vi "SRX_Config Voltage Output.vi"(8 "Error":errorcluster, 9 "Output Config":T1={"Invert?"=FALSE, "Neutral Mode"=enum."Override to Coast", "Deadband (-1to1)"=0.0, "Ramp Time Off to Full (S)"=0.0, "Peak  (-1to1)"={"Forward"=1.0, "Reverse"=-1.0}, "Nominal  (-1to1)"={"Forward"=0.0, "Reverse"=0.0}}, 11 "PhoenixMotorControlDevRef":T4={"DeviceStatus"={"status"=FALSE, "code"=0, "source"=""}, "Type"=enum."PWM", "PWM"={"PWM Channel"=enum."PWM 1", "DeadBand"={"Name"="", "maxPositivePwm"=0, "minPositivePwm"=0, "centerPwm"=0, "maxNegativePwm"=0, "minNegativePwm"=0, "angularRange"=0}}, "CAN"={"Device Number"=0, "SetOutput VI Ref"=variant(enum8{"Percent VBus", "Current", "Speed", "Position", "Voltage"} enum."Percent VBus"), "GetOutput VI Ref"=variant(refnum<k1> refnum), "Enable VI Ref"=variant(dbl 12.0), "Disable VI Ref"=variant(enum8{"Percent VBus", "Speed", "Position", "Slave", "Unchanged / Invalid", "Voltage Compensation", "Current", "Motion Profile"} enum."Percent VBus"), "Data"=variant}, "Invert"=FALSE, "DIO PWM"={"PWM \"Enable\" Channel"=enum."Invalid", "DIOChannel"=enum."Invalid", "PWM Rate"=0.0}}) -> (0 "Error Out":errorcluster, 3 "PhoenixMotorControlDevRef Out":T4={"DeviceStatus"={"status"=FALSE, "code"=0, "source"=""}, "Type"=enum."PWM", "PWM"={"PWM Channel"=enum."PWM 1", "DeadBand"={"Name"="", "maxPositivePwm"=0, "minPositivePwm"=0, "centerPwm"=0, "maxNegativePwm"=0, "minNegativePwm"=0, "angularRange"=0}}, "CAN"={"Device Number"=0, "SetOutput VI Ref"=variant(enum8{"Percent VBus", "Current", "Speed", "Position", "Voltage"} enum."Percent VBus"), "GetOutput VI Ref"=variant(refnum<k1> refnum), "Enable VI Ref"=variant(dbl 12.0), "Disable VI Ref"=variant(enum8{"Percent VBus", "Speed", "Position", "Slave", "Unchanged / Invalid", "Voltage Compensation", "Current", "Motion Profile"} enum."Percent VBus"), "Data"=variant}, "Invert"=FALSE, "DIO PWM"={"PWM \"Enable\" Channel"=enum."Invalid", "DIOChannel"=enum."Invalid", "PWM Rate"=0.0}})   [LabVIEW 2017]
uses:
  <vilib>/Rock Robotics/WPI/MotorControl/WPI_MotorControlDeviceRef.ctl
  <vilib>/Rock Robotics/WPI/MotorControl/WPI_MotorControlType.ctl
  <vilib>/Rock Robotics/SystemInterfaces/DIO/FPGA_DIOPWMChannel.ctl
  <vilib>/Rock Robotics/WPI/PWM/WPI_PWMDeadband.ctl
  <vilib>/Rock Robotics/SystemInterfaces/DIO/FPGA_DIOChannel.ctl
  TypeDefs SRX/Cluster_SRX_Config Voltage Output.ctl
  System Drivers/Phoenix-LabVIEW/Motor Controller/Controls/CTRE_Phoenix_MotorControl_NeutralMode.ctl
  TypeDefs SRX/Cluster_SRX_Forward and Reverse.ctl
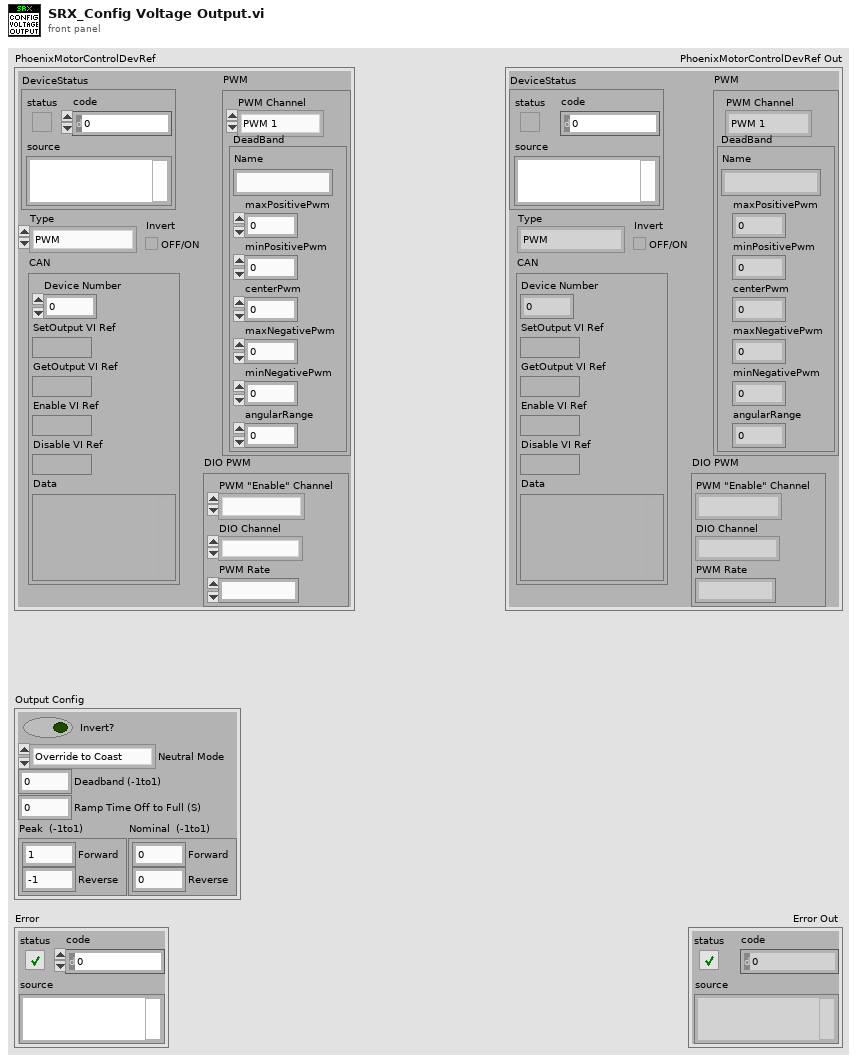
[diagram p1: front panel]
types:
  T1 = typedef "Cluster_SRX_Config Voltage Output.ctl" = cluster{"Invert?":bool, "Neutral Mode":T2, "Deadband (-1to1)":dbl, "Ramp Time Off to Full (S)":dbl, "Peak  (-1to1)":T3, "Nominal  (-1to1)":T3}
  T2 = typedef "CTRE_Phoenix_MotorControl_NeutralMode.ctl" = enum8{"EEPROMSetting", "Override to Coast", "Override to Brake"}
  T3 = typedef "Cluster_SRX_Forward and Reverse.ctl" = cluster{"Forward":dbl, "Reverse":dbl}
  T4 = typedef "WPI_MotorControlDeviceRef.ctl" = cluster{"DeviceStatus":errorcluster, "Type":T5, "PWM":cluster{"PWM Channel":T6, "DeadBand":T7}, "CAN":cluster{"Device Number":u8, "SetOutput VI Ref":variant, "GetOutput VI Ref":variant, "Enable VI Ref":variant, "Disable VI Ref":variant, "Data":variant}, "Invert":bool, "DIO PWM":cluster{"PWM \"Enable\" Channel":T6, "DIOChannel":T8, "PWM Rate":dbl}}
  T5 = typedef "WPI_MotorControlType.ctl" = enum16{"PWM", "CAN", "DIO PWM"}
  T6 = typedef "FPGA_DIOPWMChannel.ctl" = enum8{"PWM 0", "PWM 1", "PWM 2", "PWM 3", "PWM 4", "PWM 5", "PWM 6", "PWM 7", "PWM 8", "PWM 9", "PWM MXP 0", "PWM MXP 1", "PWM MXP 2", "PWM MXP 3", "PWM MXP 4", "PWM MXP 5", "PWM MXP 6", "PWM MXP 7", "PWM MXP 8", "PWM MXP 9", "Invalid"}
  T7 = typedef "WPI_PWMDeadband.ctl" = cluster{"Name":string, "maxPositivePwm":i32, "minPositivePwm":i32, "centerPwm":i32, "maxNegativePwm":i32, "minNegativePwm":i32, "angularRange":u16}
  T8 = typedef "FPGA_DIOChannel.ctl" = enum8{"DIO 0", "DIO 1", "DIO 2", "DIO 3", "DIO 4", "DIO 5", "DIO 6", "DIO 7", "DIO 8", "DIO 9", "DIO MXP 0", "DIO MXP 1", "DIO MXP 2", "DIO MXP 3", "DIO MXP 4", "DIO MXP 5", "DIO MXP 6", "DIO MXP 7", "DIO MXP 8", "DIO MXP 9", "DIO MXP 10", "DIO MXP 11", "DIO MXP 12", "DIO MXP 13", "DIO MXP 14", "DIO MXP 15", "SPI Port CS1", "SPI Port CS2", "SPI Port CS3", "SPI Port MISO", "SPI Port MOSI", "Invalid"}
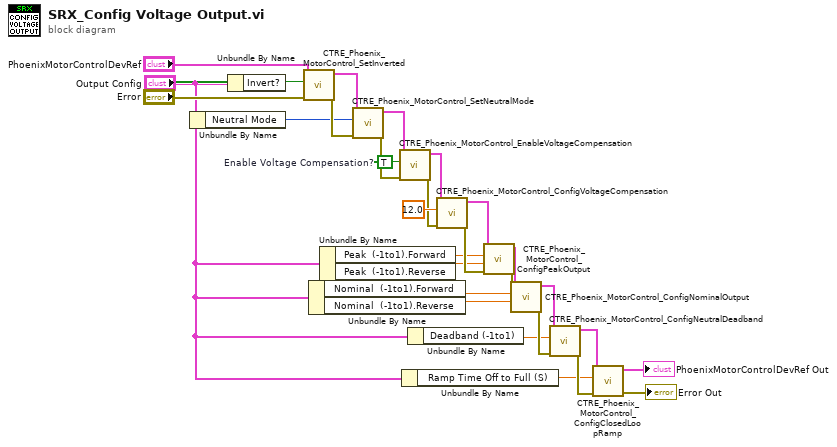
[diagram p0: block diagram]
diagram:
  w20 = TRUE  # Enable Voltage Compensation?
  n1 = Unbundle By Name("Output Config") -> ("Neutral Mode"=w8:T2)
  n2 = Unbundle By Name("Output Config") -> ("Invert?"=w9:bool)
  n3 = call "CTRE_Phoenix_MotorControl_SetInverted.vi"("error in (no error)"="Error", "Invert?"=w9, "PhoenixMotorControlDevRef"="PhoenixMotorControlDevRef") -> ("error out"=w11:errorcluster, "PhoenixMotorControlDevRef"=w27:T4)  [unwired: 7 in]
  n4 = Unbundle By Name("Output Config") -> ("Nominal  (-1to1).Forward"=w5:dbl, "Nominal  (-1to1).Reverse"=w4:dbl)
  n5 = Unbundle By Name("Output Config") -> ("Peak  (-1to1).Forward"=w6:dbl, "Peak  (-1to1).Reverse"=w7:dbl)
  n6 = call "CTRE_Phoenix_MotorControl_SetNeutralMode.vi"("error in (no error)"=w11, "Motor Control Neutral Mode"=w8, "PhoenixMotorControlDevRef"=w27) -> ("error out"=w12:errorcluster, "PhoenixMotorControlDevRef"=w26:T4)  [unwired: 7 in]
  n7 = call "CTRE_Phoenix_MotorControl_EnableVoltageCompensation.vi"("error in (no error)"=w12, "Enable Voltage Compensation?"=w20, "PhoenixMotorControlDevRef"=w26) -> ("error out"=w13:errorcluster, "PhoenixMotorControlDevRef"=w25:T4)  [unwired: 7 in]
  n8 = Unbundle By Name("Output Config") -> ("Ramp Time Off to Full (S)"=w1:dbl)
  n9 = Unbundle By Name("Output Config") -> ("Deadband (-1to1)"=w3:dbl)
  n10 = call "CTRE_Phoenix_MotorControl_ConfigVoltageCompensation.vi"("error in (no error)"=w13, "Saturation Voltage"=12.0, "PhoenixMotorControlDevRef"=w25) -> ("error out"=w14:errorcluster, "PhoenixMotorControlDevRef"=w24:T4)  [unwired: 7 in]
  n11 = call "CTRE_Phoenix_MotorControl_ConfigPeakOutput.vi"("error in (no error)"=w14, "Reverse Peak Percent Output"=w7, "Forward Peak Percent Output"=w6, "PhoenixMotorControlDevRef"=w24) -> ("error out"=w15:errorcluster, "PhoenixMotorControlDevRef"=w23:T4)  [unwired: 6 in]
  n12 = call "CTRE_Phoenix_MotorControl_ConfigNominalOutput.vi"("error in (no error)"=w15, "Reverse Nominal Percent Output"=w4, "Forward Nominal Percent Output"=w5, "PhoenixMotorControlDevRef"=w23) -> ("error out"=w16:errorcluster, "PhoenixMotorControlDevRef"=w22:T4)  [unwired: 6 in]
  n13 = call "CTRE_Phoenix_MotorControl_ConfigNeutralDeadband.vi"("error in (no error)"=w16, "Percent Deadband"=w3, "PhoenixMotorControlDevRef"=w22) -> ("error out"=w17:errorcluster, "PhoenixMotorControlDevRef"=w21:T4)  [unwired: 7 in]
  n14 = call "CTRE_Phoenix_MotorControl_ConfigClosedLoopRamp.vi"("error in (no error)"=w17, "secondsFromNeutralToFull"=w1, "PhoenixMotorControlDevRef"=w21) -> ("error out"=→"Error Out":errorcluster, "PhoenixMotorControlDevRef"=→"PhoenixMotorControlDevRef Out":T4)  [unwired: 7 in]
